vi "Power Test.vi"(11 "Amplitude":dbl(slide)=10.0 scale=0.0..10.0) -> (1 "frequency":dbl, 3 "tdms file path":string)   [LabVIEW 2018]
uses:
  <vilib>/measure/matone.llb/Extract Single Tone Information N Chan.vi
  <vilib>/Waveform/WDTOps.llb/WDT Number of Waveform Samples DBL.vi
  <vilib>/measure/NI_MAPro.lvlib
panel:
  out "number of samples":i32
  out "Waveform Graph":dynamicdata(graph)
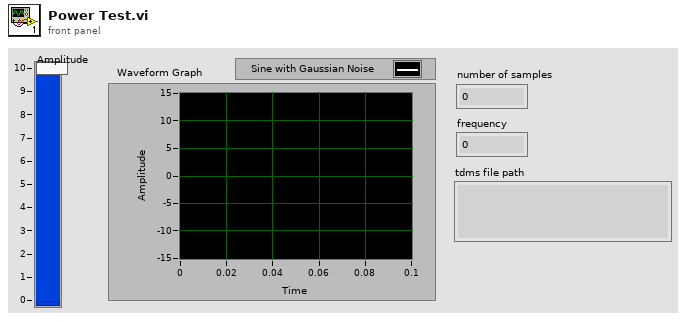
[diagram p1: front panel]
types:
  T1 = enum16{"open", "open or create", "create or replace", "create", "open (read-only)"}
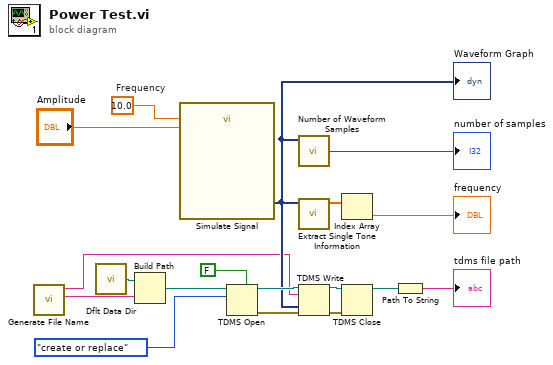
[diagram p0: block diagram]
diagram:
  w14 = 10.0  # Frequency
  n1 = call "Generate File Name.vi"() -> ("file name"=w2:string, "system"=w1:string)  [unwired: 9 in]
  n2 = call <vilib>:"Dflt Data Dir.vi"() -> ("App:Default Data Directory"=w3:path)
  n3 = Build Path(base path=w3, name or relative path=w2) -> (appended path=w5:path)
  n4 = call "Simulate Signal"("Frequency"=w14, "Amplitude"="Amplitude") -> ("Sine with Gaussian Noise"=w11:dynamicdata)  [unwired: 12 in, 1 out]
  "Waveform Graph" <- w11
  n5 = TDMS Open(5:FALSE ("create index file? (T)"), 10:T1."create or replace" ("operation (0:open)"), 11:w5) -> (0:w7:errorcluster, 3:w12:refnum<k34>)  [unwired: 4 in]
  n6 = call-poly <vilib>:"Number of Waveform Samples.vi"("waveform in"=w11) -> ("number of samples"=→"number of samples":i32)  [unwired: 8 in, 2 out]
  n7 = call-poly <vilib>:"Extract Single Tone Information.vi"("time signals in"=w11) -> ("detected frequencies"=w16:dbl[])  [unwired: 5 in, 5 out]
  n8 = TDMS Write(0:w12, 5:w1, 9:w11, 11:w7) -> (4:w10:refnum<k34>, 15:w9:errorcluster)  [unwired: 2 in, 2 out]
  n9 = Index Array(array=w16) -> (element=→"frequency":dbl)  [unwired: 1 in]
  n10 = TDMS Close(8:w9, 11:w10) -> (3:w4:path)  [unwired: 1 out]
  n11 = Path To String(path=w4) -> (string=→"tdms file path":string)
